vi "GEA2 Serial File Com Config.vi"(0 "file path (dialog if empty)":path=path "c:/work/ComArray.ini", 7 "Read/Write?":bool=TRUE) -> (6 "Com Array Out":u8[](array[numeric])=[100, 2, 3, 4, 5, 6, 7, 8, 9, 10, 11, 12, 13, 14, 15, 16, 17, 18, 19, 20, 21, 22, 23, 24, 25, 26, 27, 28, 29, 30, 31, 32, 33, 34, 35, 36, 37, 38, 39, 40, 41, 42, 43, 44, 45, 46, 47, 48, 49, 50, 51, 52, 53, 54, 55, 56], 8 "Station Labels":string[](array[string]))   [LabVIEW 2014]
uses:
  <vilib>/Utility/file.llb/Read From Spreadsheet File (I64).vi
  <vilib>/Utility/file.llb/Write To Spreadsheet File (I64).vi
panel:
  in  "Station Labels to Write":string[](array[string])=["W01", "W02", "W03", "W04", "W05", "W06", "W07", "W08", "W09", "W10", "W11", "W12", "W13", "W14", "W15", "W16", "W17", "W18", "W19", "W20", "W21", "W22", "W23", "W24", "W25", "W26", "W27", "W28", "W29", "W30", "W31", "W32", "W33", "W34", "W35", "W36", "W37", "W38", "W39", "W40", "W41", "W42", "W43", "W44", "W45", "W46", "W47", "W48", "W49", "W50", "W51", "W52", "W53", "W54", "W55", "W56"]
  out "text":string
  in  "Com Array To Write":u8[](array[numeric])=[100, 2, 3, 4, 5, 6, 7, 8, 9, 10, 11, 12, 13, 14, 15, 16, 17, 18, 19, 20, 21, 22, 23, 24, 25, 26, 27, 28, 29, 30, 31, 32, 33, 34, 35, 36, 37, 38, 39, 40, 41, 42, 43, 44, 45, 46, 47, 48, 49, 50, 51, 52, 53, 54, 55, 56]
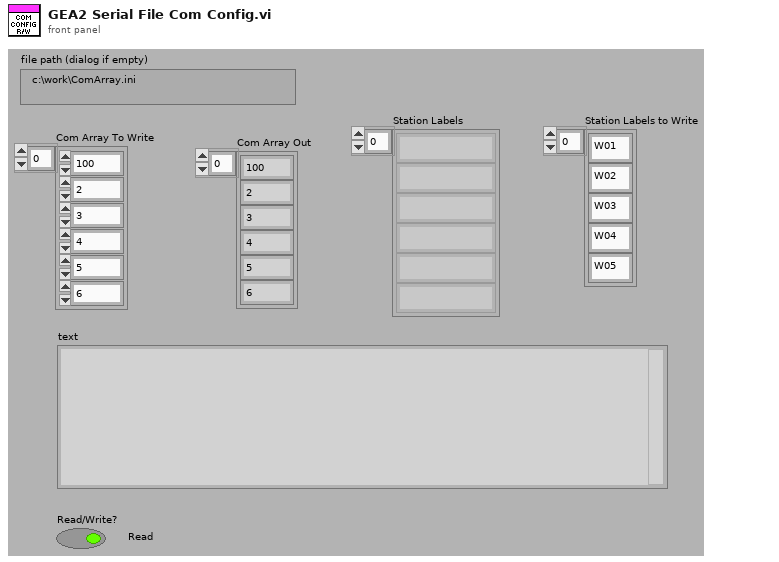
[diagram p1: front panel]
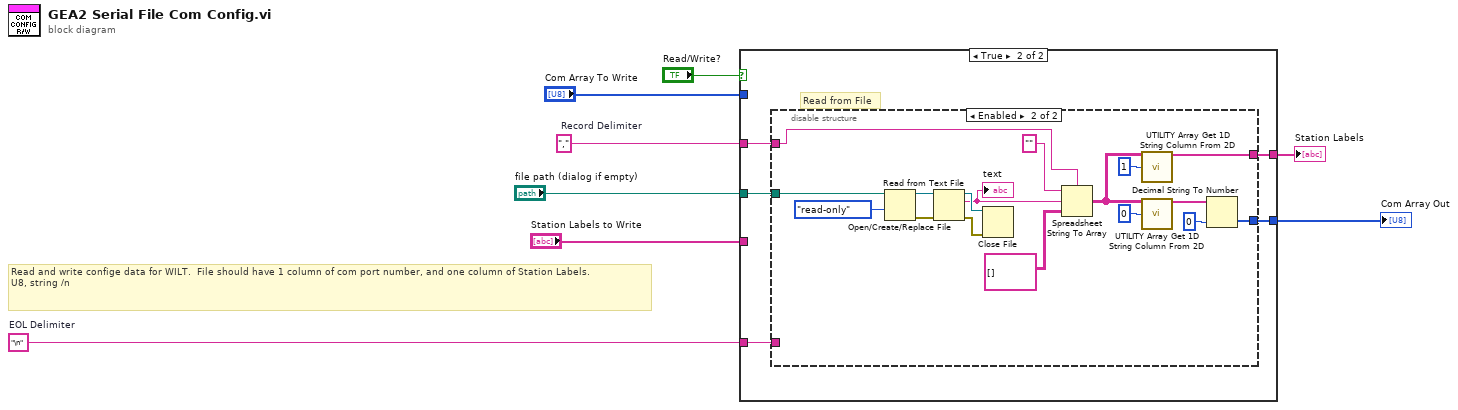
[diagram p0: block diagram]
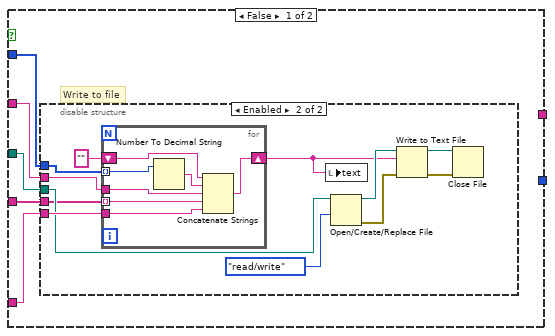
[diagram p2: hidden frame]
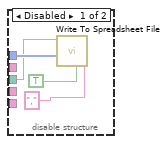
[diagram p3: hidden frame]
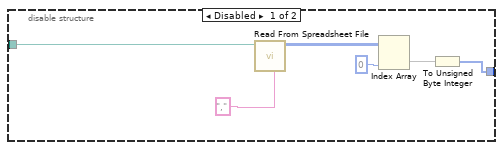
[diagram p4: hidden frame]
diagram:
  w1 = ","  # Record Delimiter
  w4 = "\n"  # EOL Delimiter
  # "Read and write confige data for WILT.  File should have 1 column of com port number, and one column of Station Labels.\nU8, string /n"
  n1 = case shown="True" "Read/Write?" {
    tunnel: "Com Array To Write" -> [w13 _]
    tunnel: "file path (dialog if empty)" -> [w12 w41]
    tunnel: [_ w40] -> w6
    tunnel: [_ w39] -> w3
    tunnel: w4 -> [w10 w38]
    tunnel: "Station Labels to Write" -> [w11 _]
    tunnel: w1 -> [w9 w37]
    frame False {
      # "Write to file"
      n2 = disable-structure shown="Enabled" {
        disable-tunnel: w13 -> [w17 w24]
        disable-tunnel: w12 -> [w16 w22]
        disable-tunnel: w11 -> [_ w20]
        disable-tunnel: w10 -> [_ w23]
        disable-tunnel: w9 -> [_ w21]
        frame Disabled {
          n3 = call-poly <vilib>:"Write To Spreadsheet File.vi"("delimiter (\\t)"="," ("delimiter (\\t)"), "transpose? (no:F)"=TRUE, "1D data"=w17, "file path (dialog if empty)"=w16) -> ()  [unwired: 4 in, 1 out]
        }
        frame Enabled {
          n4 = for {
            tunnel: w24 -> [w36] mode=indexing
            tunnel: w23 -> [w32]
            tunnel: w21 -> [w35]
            tunnel: w20 -> [w33] mode=indexing
            shift-right: [w31] -> w19
            shift-left: "" -> [w30]
            n5 = Number To Decimal String(number=w36) -> (decimal integer string=w34:string)  [unwired: 1 in]
            n6 = Concatenate Strings(w30, w34, w35, w33, w32) -> (w31:string)
          }
          n7 = local write "text"(w19) -> ()
          n8 = Open/Create/Replace File(file path (use dialog)=w22, access (0:read/write)=enum16{"read/write", "read-only", "write-only"}."read/write") -> (refnum out=w27:refnum<file>, error out=w28:errorcluster)  [unwired: 4 in, 1 out]
          n9 = Write to Text File(file (use dialog)=w27, text=w19, error in=w28) -> (refnum out=w25:refnum<file>, error out=w26:errorcluster)  [unwired: 1 in, 1 out]
          n10 = Close File(refnum=w25, error in=w26) -> ()  [unwired: 2 out]
        }
      }
    }
    frame True {
      # "Read from File"
      n11 = disable-structure shown="Enabled" {
        disable-tunnel: w41 -> [w47 w64]
        disable-tunnel: [w43 w55] -> w40
        disable-tunnel: [_ w49] -> w39
        disable-tunnel: w38 -> [_ _]
        disable-tunnel: w37 -> [_ w48]
        frame Disabled {
          n12 = call-poly <vilib>:"Read From Spreadsheet File.vi"("delimiter (\\t)"="," ("delimiter (\\t)"), "file path (dialog if empty)"=w47) -> ("all rows"=w46:i64[][])  [unwired: 5 in, 4 out]
          n13 = Index Array(array=w46, index (col)=0 ("disabled index (col)")) -> (element=w44:i64[])  [unwired: 1 in]
          n14 = To Unsigned Byte Integer(number=w44) -> (unsigned 8bit integer=w43:u8[])
        }
        frame Enabled {
          n15 = Open/Create/Replace File(file path (use dialog)=w64, access (0:read/write)=enum16{"read/write", "read-only", "write-only"}."read-only") -> (refnum out=w61:refnum<file>, error out=w62:errorcluster)  [unwired: 4 in, 1 out]
          n16 = Read from Text File(file (use dialog)=w61, error in=w62) -> (refnum out=w59:refnum<file>, text=w56:string, error out=w60:errorcluster)  [unwired: 2 in, 1 out]
          "text" <- w56
          n17 = Close File(refnum=w59, error in=w60) -> ()  [unwired: 2 out]
          n18 = Spreadsheet String To Array(delimiter (Tab)=w48, format string="", spreadsheet string=w56, array type (2D Dbl)=string[][] []) -> (array=w53:string[][])
          n19 = call "UTILITY Array Get 1D String Column From 2D.vi"("2D Array Data"=w53, "column index"=1) -> ("Column Data"=w49:string[])  [unwired: 13 in]
          n20 = call "UTILITY Array Get 1D String Column From 2D.vi"("2D Array Data"=w53, "column index"=0) -> ("Column Data"=w50:string[])  [unwired: 13 in]
          n21 = Decimal String To Number(string=w50, default (0L)=u8 0 ("default (0 I32)")) -> (number=w55:u8[])  [unwired: 1 in, 1 out]
        }
      }
    }
  }
  "Com Array Out" <- w6
  "Station Labels" <- w3
